vi "Read All Child Attributes.vi"(11 "Core Actor in":refnum<class "Core Actor.lvclass">) -> (2 "All Child Attributes":T1)   [LabVIEW 2025, in "jettl.lvlib" / "Base Actor.lvlib" / "Core Actor.lvclass"]
uses:
  Core Actor.lvclass
  All Child Attributes.ctl
  Attributes/Attributes.lvclass
  Core Actor.lvclass/Core Actor.ctl
  jettl.lvlib
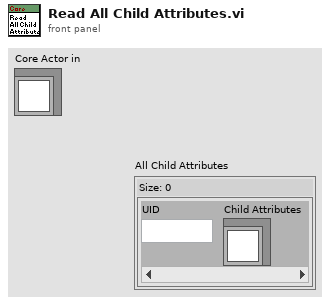
[diagram p1: front panel]
types:
  T1 = typedef "jettl.lvlib/All Child Attributes.ctl" = map{string, refnum<class "Attributes.lvclass">}
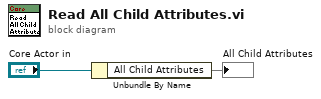
[diagram p0: block diagram]
diagram:
  n1 = Unbundle By Name("Core Actor in") -> ("All Child Attributes"=→"All Child Attributes":T1)
